vi "Order Tracking Mangitude and Phase (Analog Tacho, DAQmx) .vi"() -> ()   [LabVIEW 2017]
doc: "This VI demonstrates how to compute order magnitude and phase. This VI uses DAQmx VIs to acquire sound or vibration signals and an analog tachometer signal and displays order magnitude and phase results continuously. \n\n<B>INSTRUCTIONS</B>:\n1. On the <B>DAQ Configurations</B> page, specify the <B>sample rate</B>, <B>samples per channel</B>, device and channel configurations, and tachometer channel information.\n2. On the <B>Magnitude and Phase</B> page, specify the <B>orders to compute</B>, <B>view</B>, <B>magnitude view</B>, and <B>x-axis selection</B> to get the desired order magnitude and phase display. \n3. Run the VI.\n4. On the <B>Magnitude and Phase</B> page, select the signal of interest in the <B>select channel</B> control.\n\n<B>VIs USED IN THIS EXAMPLE</B>:\n1. SVL Scale Voltage to EU.vi\n2. OAT Analog Tacho Process.vi\n3. OAT Convert to Even Angle Signal.vi\n4. OAT Order Magnitude and Phase.vi\n5. SVL Unit Conversion.vi"
uses:
  <vilib>/addons/Sound and Vibration/Order Analysis/Example Support/sub VIs/OAXML_DSA DAQ Config.ctl
  <vilib>/addons/_NISVFA/_Shared subVIs/Controls/svc_Engineering Units Text Ring.ctl
  <vilib>/addons/Sound and Vibration/Order Analysis/Utility/SubVIs/oa_Buffer Settings.ctl
  <vilib>/DAQmx/read.llb/DAQmx Read (Analog 1D Wfm NChan NSamp).vi
  <vilib>/addons/Sound and Vibration/Order Analysis/Utility/OAT Output Buffered Data (XY, N Chan).vi
  <vilib>/addons/Sound and Vibration/Order Analysis/Utility/OAT Even Time or Speed Segment (XY, 1D Array).vi
  <vilib>/addons/_NISVFA/_Spectrum Processing/SVFA Unit Conversion (XY) (1 Ch - M Orders).vi
  <vilib>/addons/Sound and Vibration/Order Analysis/Resample Order Tracking/OAT Order Magnitude and Phase (Even Angle Signal, N Channels).vi
  <vilib>/addons/Sound and Vibration/Order Analysis/Resample Order Tracking/OAT Convert to Even Angle Signal (N Channels).vi
  <vilib>/addons/Sound and Vibration/Order Analysis/Tach Process/OAT Analog Tacho Process (1 Tacho).vi
  <vilib>/DAQmx/miscellaneous.llb/DAQmx Fill In Error Info.vi
  <vilib>/addons/Sound and Vibration/Order Analysis/Tach Process/SoundVib_TachProcess.lvlib
  <vilib>/addons/Sound and Vibration/Order Analysis/Utility/SoundVib_OAUtility.lvlib
  <vilib>/addons/Sound and Vibration/Order Analysis/Resample Order Tracking/SoundVib_OrderTracking.lvlib
panel:
  in  "stop":bool
  in  "Tab Control":T1(tab)
  in  "samples per channel":i32=5000
  in  "slope (Rising)":u16(ring) items=["Rising", "Falling"]
  in  "threshold (auto)":dbl=inf format="%.2f"
  in  "pulse / rev":i32=1
  in  "sample rate [samples/s]":dbl=10000.0
  in  "Min Value":dbl=-5.0 format="%0.2f"
  in  "Max Value":dbl=5.0 format="%0.2f"
  in  "DAQ Config":T2 {"pregain" format="%.2f"; "IEPE" items=["On", "Off", "None"]; "coupling" items=["DC", "AC"]; "engineering units" items=["custom..."=0, "V"=1, "A"=21, "C"=30, "pC"=31, "s"=32, "-"=29, "Pa"=2, "N"=20, "g"=3, "m/s^2"=4, "m/s"=5, "m"=6, "mm/s"=12, "mm"=13, "micron/s"=14, "micron"=15, "in/s^2"=7, "in/s"=8, "in"=9, "mil/s"=10, "mil"=11, "rad/s^2"=16, "rad/s"=17, "rad"=18, "deg/s^2"=26, "deg/s"=27, "deg"=28, "RPM"=22, "cycle/s^2"=23, "Hz"=24, "cycle"=25, "strain"=19]; "sensor sensitivity (mV/EU)" format="%.2f"; "dB reference" format="%.1e"}
  in  "tachometer channel":tag
  out "Speed profile":cluster{"time [s]":dbl[], "speed [rpm]":dbl[]}(graph)
  out "Acquired waveform":waveform(dbl)[](graph)
  in  "view":T4={"dB on? (F)"=FALSE, "unwrap phase? (T)"=TRUE, "unit in degree? (T)"=TRUE}
  in  "magnitude view":enum16{"no change", "rms", "peak", "peak-peak"}(ring)
  in  "X axis selection":u16(ring) items=["Time", "Revolution", "RPM"]
  in  "bandwidth [order]":dbl=1.0 format="%.2f"
  in  "orders to compute":dbl[](array[numeric])=[1.0] format="%.2f"
  in  "select channel":u16(ring)
  out "Phase":cluster{"time/rev/rpm":dbl[], "phase":dbl[]}[](graph)
  out "Magnitude":T5(graph)
  in  "segment settings":cluster{"start":dbl, "end":dbl, "step size":dbl} {"step size" format="%.2f"; "end" min=0.0 format="%.2f"; "start" min=0.0 format="%.2f"}
  # "Select Help»Show Context Help \nand move the cursor over the VI \nicon for more information."
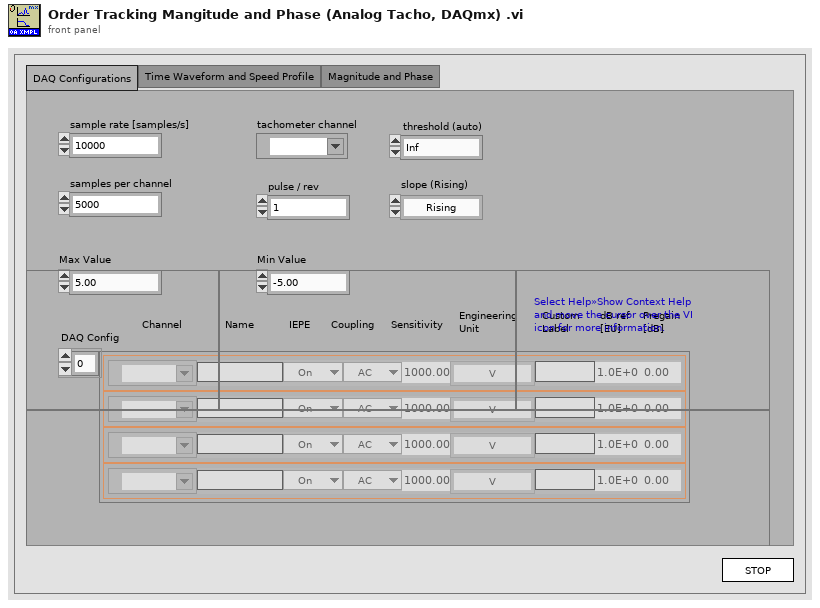
[diagram p1: front panel]
types:
  T1 = enum32{"DAQ Configurations", "Time Waveform and Speed Profile", "Magnitude and Phase"}
  T2 = typedef "OAXML_DSA DAQ Config.ctl" = cluster{"name":string, "channel":tag, "coupling":u16, "dB reference":sgl, "sensor sensitivity (mV/EU)":dbl, "engineering units":T3, "IEPE":u16, "custom label":string, "pregain":sgl}[]
  T3 = typedef "svc_Engineering Units Text Ring.ctl" = u16
  T4 = cluster{"dB on? (F)":bool, "unwrap phase? (T)":bool, "unit in degree? (T)":bool}
  T5 = cluster{"time/rev/rpm":dbl[], "magnitude":dbl[]}[]
  T6 = typedef "svc_Channel Info.ctl" = cluster{"sensor sensitivity":dbl, "engineering units":T3, "dB reference":dbl, "custom label":string, "weighting filter":T7, "pregain":dbl}
  T7 = typedef "svc_Weighting Filter Text Ring.ctl" = u16
  T8 = typedef "SoundVib_OAUtility.lvlib/oa_Buffer Settings.ctl" = cluster{"buffer size":dbl, "buffer unit":enum16{"s", "revolution", "# of samples"}}
  T9 = typedef "SoundVib_TachProcess.lvlib/speed profile.ctl" = cluster{"time [s]":dbl[], "speed [RPM]":dbl[]}
  T10 = typedef "svc_Resampled Channel Info.ctl" = cluster{"channel name":string, "description":string, " channel info":T6}
  T11 = typedef "OAT Position Info.ctl" = cluster{"positions [s]":dbl[], "samples/rev":dbl}
  T12 = cluster{"x unit":string, "magnitude unit":string, "phase unit":string}[]
  T13 = cluster{"time/rev/rpm":dbl[], "magnitude":dbl[]}[][]
  T14 = typedef "svc_Spectrum Info.ctl" = cluster{"channel name":string, "description":string, "x-axis units":T15, "spectral info":cluster{"spectrum type":T16, "linear/dB":enum16{"linear", "dB"}, "window":u16, "window size":i32, "FFT size":i32}, "engineering units":T3, "custom label":string, "dB reference [EU]":dbl, "peak units":enum16{"rms", "peak", "peak-peak"}, "weighting filter":T7, "spectral density?":bool, "unit label":string, "spectrum skewed?":bool, "complimentary spectrum units":T17}
  T15 = typedef "svc_X-Axis Units.ctl" = u16
  T16 = typedef "svc_Spectrum Type.ctl" = enum16{"FFT Spectrum [complex]", "Amplitude [Magnitude]", "Power [Magnitude^2]", "Cross Spectrum [complex]", "Frequency Response [Complex]"}
  T17 = typedef "svc_Complimentary Spectrum Units.ctl" = enum16{"none", "radians", "degrees", "cycles", "imaginary"}
  T18 = cluster{"x unit":string, "magnitude unit":string, "phase unit":string}
  T19 = cluster{"linear/dB":enum16{"no change", "linear", "dB"}, "dB reference (0: no change)":dbl, "power/magnitude":enum16{"no change", "power", "magnitude"}, "view":enum16{"no change", "rms", "peak", "peak-peak"}}
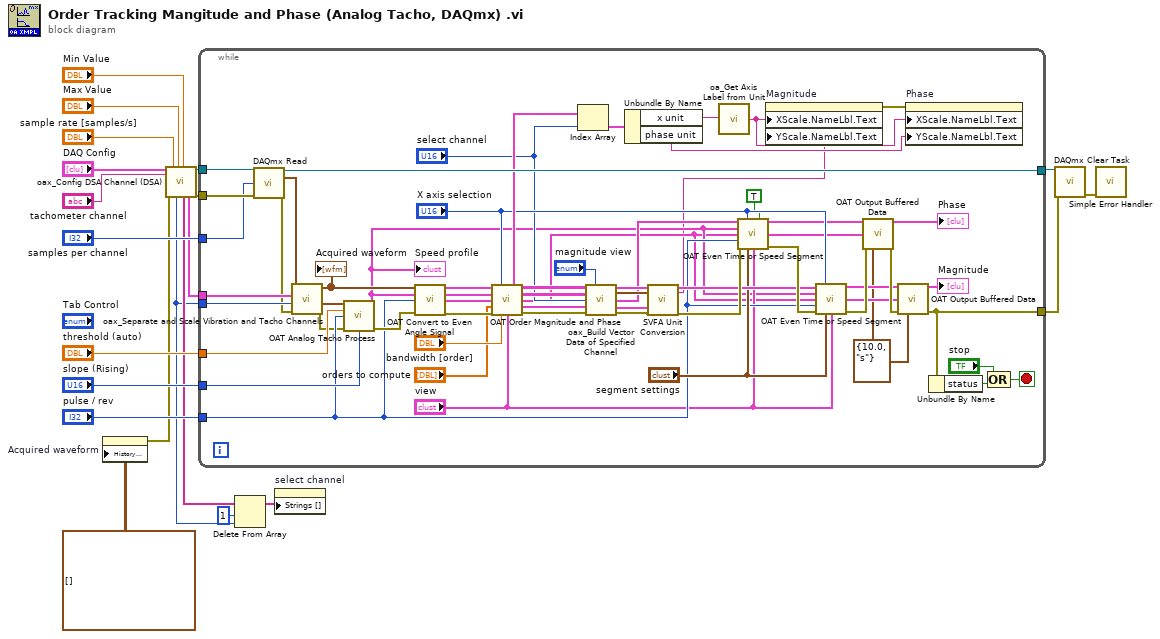
[diagram p0: block diagram]
diagram:
  n1 = property on="Acquired waveform" class="WFChart (strict)"("History Data"=waveform(dbl)[][] []) -> (error out=w2:errorcluster)  [unwired: 2 in, 1 out]
  n2 = call <vilib>:"oax_Config DSA Channel (DSA).vi"("DAQ Config"="DAQ Config", "tachometer channel"="tachometer channel", "error in (no error)"=w2, "sample rate [samples/s]"="sample rate [samples/s]", "max value"="Max Value", "min value"="Min Value") -> ("channel name"=w12:string[], "channel info"=w11:T6[], "task out"=w9:refnum<k21>, "tacho channel index"=w8:i32, "error out"=w10:errorcluster)  [unwired: 9 in]
  n3 = while {
    tunnel: w9 -> [w82]
    tunnel: [w70] -> w14
    tunnel: "pulse / rev" -> [w49]
    tunnel: "slope (Rising)" -> [w79]
    tunnel: "threshold (auto)" -> [w80]
    tunnel: w11 -> [w66]
    tunnel: "samples per channel" -> [w69]
    tunnel: w8 -> [w65]
    tunnel: w10 -> [w81]
    tunnel: [w38] -> w21
    stop <- w77 stop-if-true
    w37 = T8 {"buffer size"=10.0, "buffer unit"=enum."s"} ("buffer settings")
    n4 = call-poly <vilib>:"DAQmx Read.vi"("task/channels in"=w82, "number of samples per channel"=w69, "error in"=w81) -> ("task out"=w70:refnum<k21>, "data"=w67:waveform(dbl)[], "error out"=w26:errorcluster)  [unwired: 10 in]
    n5 = call <vilib>:"oax_Separate and Scale Vibration and Tacho Channels.vi"("error in (no error)"=w26, "tacho channel index"=w65, "channel info in"=w66, "waveform in"=w67) -> ("error out"=w34:errorcluster, "tacho out"=w35:waveform(dbl), "noise or vibration waveform out"=w36:waveform(dbl)[])  [unwired: 5 in]
    "Acquired waveform" <- w36
    n6 = call-poly <vilib>:"OAT Analog Tacho Process.vi"("analog tacho signal"=w35, "threshold (auto)"=w80, "pulse/revolution (1)"=w49, "error in (no error)"=w34, "slope (Rising)"=w79) -> ("speed profile"=w25:T9, "error out"=w68:errorcluster)  [unwired: 6 in, 3 out]
    "Speed profile" <- w25
    n7 = call-poly <vilib>:"OAT Convert to Even Angle Signal.vi"("scaled signals [EU]"=w36, "speed profile"=w25, "pulse/revolution (1)"=w49, "error in (no error)"=w68) -> ("even-angle signals"=w75:cluster{"r0":dbl, "dr":dbl, "Y":dbl[]}[], "even-angle channel info"=w74:T10[], "even-angle position info"=w73:T11, "error out"=w71:errorcluster)  [unwired: 7 in, 1 out]
    n8 = call-poly <vilib>:"OAT Order Magnitude and Phase.vi"("even-angle signals"=w75, "x-axis selection"="X axis selection", "even-angle channel info"=w74, "even-angle position info"=w73, "orders to compute (1.0)"="orders to compute", "error in (no error)"=w71, "bandwidth [order]"="bandwidth [order]", "view"="view") -> ("unit labels"=w56:T12, "magnitudes [RMS]"=w64:T13, "phases [phase lag]"=w63:cluster{"time/rev/rpm":dbl[], "phase":dbl[]}[][], "magnitude/phase position info"=w24:T11, "magnitudes info"=w62:T14[], "error out"=w29:errorcluster)  [unwired: 2 in]
    n9 = Index Array(array=w56, index="select channel") -> (element=w55:T18)
    n10 = call <vilib>:"oax_Build Vector Data of Specified Channel.vi"("magnitudes [RMS]"=w64, "magnitude view"="magnitude view", "phase [phase lag]"=w63, "select channel"="select channel", "magnitudes info"=w62, "error in (no error)"=w29) -> ("magnitudes"=w59:T5, "desired scaling"=w58:T19, "phase"=w54:cluster{"time/rev/rpm":dbl[], "phase":dbl[]}[], "magnitude info"=w57:T14, "error out"=w27:errorcluster)  [unwired: 5 in]
    n11 = Unbundle By Name(w55) -> ("x unit"=w32:string, "phase unit"=w30:string)
    n12 = call-poly <vilib>:"SVFA Unit Conversion.vi"("magnitudes"=w59, "desired scaling"=w58, "magnitude info in"=w57, "error in (no error)"=w27) -> ("converted magnitudes"=w51:T5, "unit label"=w22:string, "error out"=w53:errorcluster)  [unwired: 12 in, 1 out]
    n13 = call <vilib>:"oa_Get Axis Label from Unit.vi"("Unit"=w32) -> ("Label"=w31:string)  [unwired: 4 in]
    n14 = call-poly <vilib>:"OAT Even Time or Speed Segment.vi"("XY signals"=w54, "x-axis selection"="X axis selection", "phase input? (F)"=TRUE, "speed profile"=w25, "position info"=w24, "pulse/revolution (1)"=w49, "error in (no error)"=w53, "segment settings"="segment settings", "view info"="view") -> ("XY signals out"=w46:cluster{"X":dbl[], "Y":dbl[]}[], "position info out"=w44:T11, "error out"=w52:errorcluster)  [unwired: 2 in, 2 out]
    n15 = property on="Magnitude" class="XYGraph (strict)"("XScale.NameLbl.Text"=w31, "YScale.NameLbl.Text"=w22) -> (error out=w33:errorcluster)  [unwired: 2 in, 1 out]
    n16 = call-poly <vilib>:"OAT Even Time or Speed Segment.vi"("XY signals"=w51, "x-axis selection"="X axis selection", "speed profile"=w25, "position info"=w24, "pulse/revolution (1)"=w49, "error in (no error)"=w52, "segment settings"="segment settings", "view info"="view") -> ("XY signals out"=w41:cluster{"X":dbl[], "Y":dbl[]}[], "position info out"=w40:T11, "error out"=w45:errorcluster)  [unwired: 3 in, 2 out]
    n17 = call-poly <vilib>:"OAT Output Buffered Data.vi"("XY signals"=w46, "position info"=w44, "error in (no error)"=w45, "buffer settings"=w37) -> ("buffered XY signals"=→"Phase":cluster{"X":dbl[], "Y":dbl[]}[], "error out"=w42:errorcluster)  [unwired: 9 in, 1 out]
    n18 = call-poly <vilib>:"OAT Output Buffered Data.vi"("XY signals"=w41, "position info"=w40, "error in (no error)"=w42, "buffer settings"=w37) -> ("buffered XY signals"=→"Magnitude":cluster{"X":dbl[], "Y":dbl[]}[], "error out"=w38:errorcluster)  [unwired: 9 in, 1 out]
    n19 = property on="Phase" class="XYGraph (strict)"(error in=w33, "XScale.NameLbl.Text"=w31, "YScale.NameLbl.Text"=w30) -> ()  [unwired: 1 in, 2 out]
    n20 = Unbundle By Name(w38) -> ("status"=w78:bool)
    n21 = Compound Arithmetic op=OR("stop", w78) -> (w77:bool)
  }
  n22 = Delete From Array(array=w12, length=1 ("index"), index=w8) -> (array with subset deleted=w13:string[])  [unwired: 1 out]
  n23 = property on="select channel" class="Ring (strict)"("Strings []"=w13) -> ()  [unwired: 2 in, 2 out]
  n24 = call <vilib>:"DAQmx Clear Task.vi"("task in"=w14, "error in"=w21) -> ("error out"=w16:errorcluster)  [unwired: 13 in]
  n25 = call <vilib>:"Simple Error Handler.vi"("error in (no error)"=w16) -> ()  [unwired: 4 in, 5 out]
